vi "Read Content.vi"(8 "Error In":errorcluster, 11 "Root In":refnum<class "Root.lvclass">) -> (0 "Error Out":errorcluster, 2 "Content":string, 3 "Root Out":refnum<class "Root.lvclass">)   [LabVIEW 2018, in "Toolkit.lvlib" / "Nodes.lvlib" / "Root.lvclass"]
uses:
  Root.lvclass
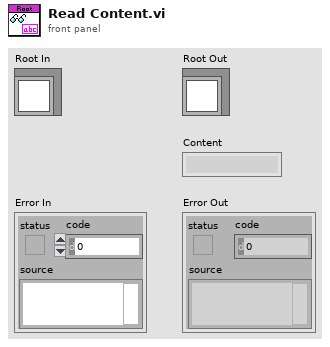
[diagram p1: front panel]
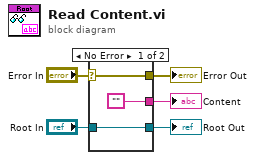
[diagram p0: block diagram]
diagram:
  n1 = case shown="No Error" "Error In" {
    selector: "Error In" -> [w8 w10]
    tunnel: [w8 w10] -> w4
    tunnel: "Root In" -> [w7 w9]
    tunnel: [w7 w9] -> w2
    tunnel: ["" _] -> w1
    frame No Error {
    }
    frame Error {
    }
  }
  "Error Out" <- w4
  "Root Out" <- w2
  "Content" <- w1
